vi "main.vi"() -> ()   [LabVIEW 2013]
doc: "使用该模板构建标准状态机设计模式。各状态执行代码并决定转移状态。将该设计模式与根据用户动作响应而执行代码的用户界面事件处理器模式相比较。同时将该设计模式与每段消息处理代码可以将零至多个新消息加入队列的队列消息处理器模式相比较。\n注：该模板的设计未遵守最新NI推荐的编程风格。请通过“创建项目”对话框（而不要采用该模板），创建基于项目的标准状态机模式的完整实现。"
uses:
  main.ctl
panel:
  in  "添加":bool
  in  "商店信息":cluster{"店名":string, "营业":bool, "位置":string}
  in  "树形":string(tree)
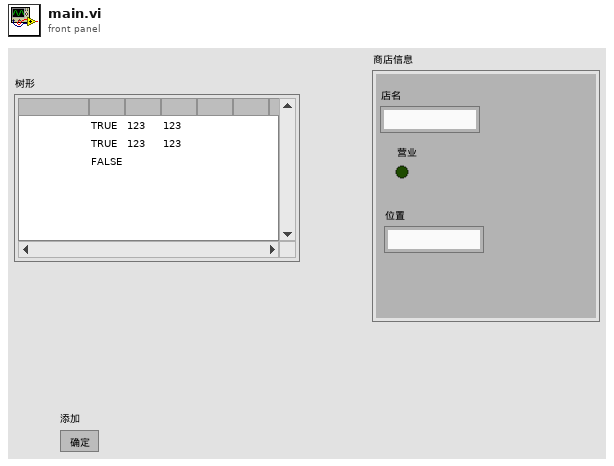
[diagram p1: front panel]
types:
  T1 = typedef "main.ctl" = enum16{"删除商店信息", "添加商店信息", "Initialize", "Stop"}
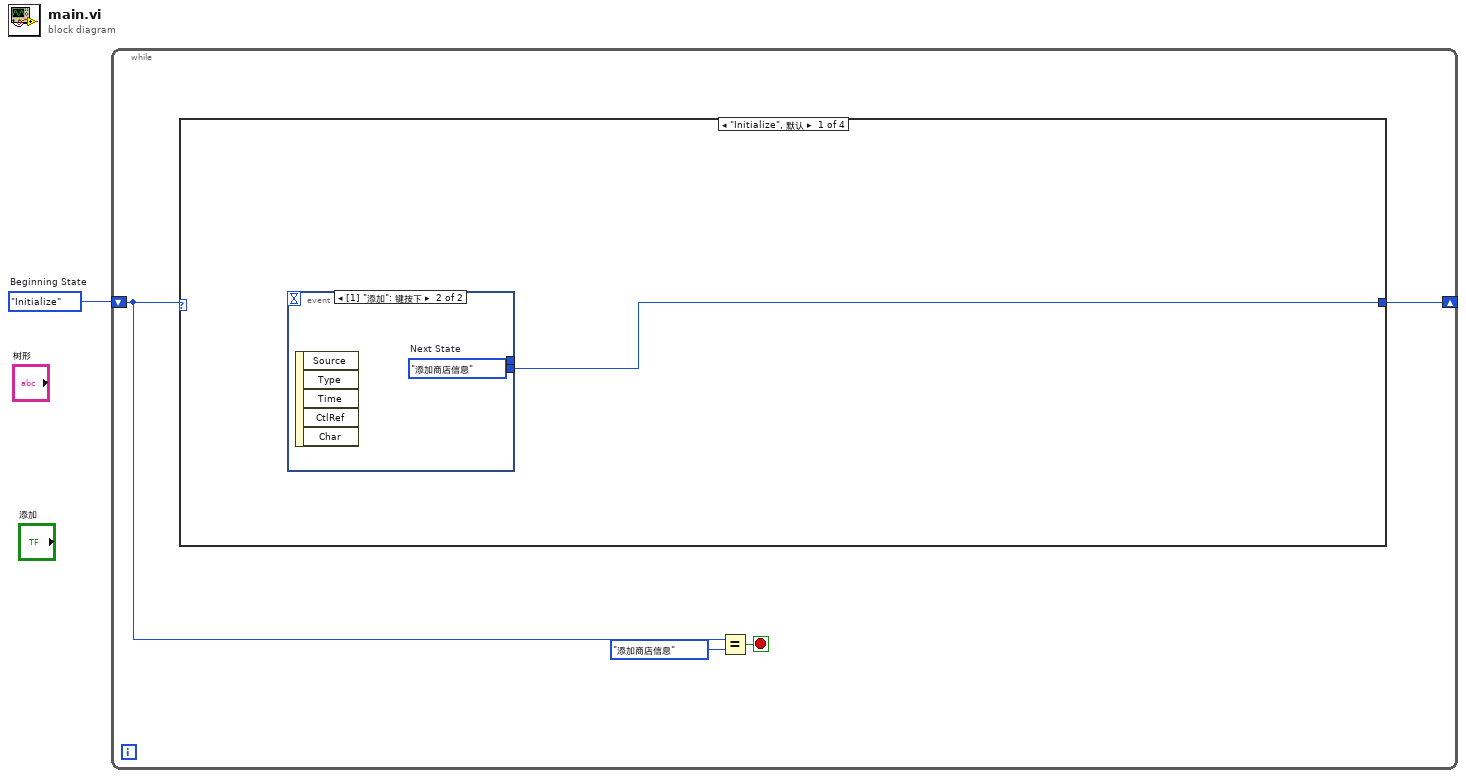
[diagram p0: block diagram]
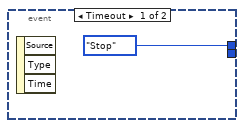
[diagram p2: hidden frame]
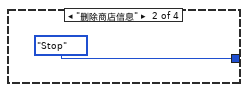
[diagram p3: hidden frame]
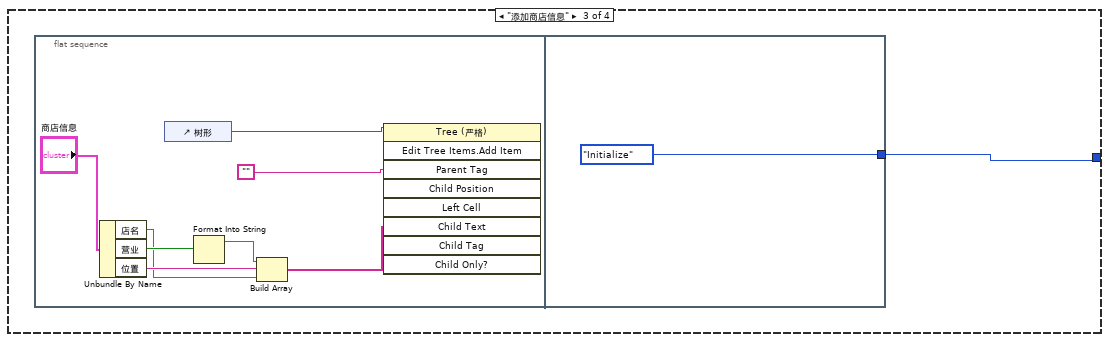
[diagram p4: hidden frame]
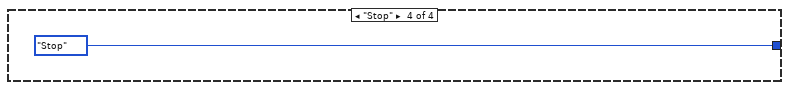
[diagram p5: hidden frame]
diagram:
  w1 = main."Initialize"  # Beginning State
  n1 = while {
    shift-right: [w2] -> _
    shift-left: w1 -> [w3]
    stop <- w5 stop-if-true
    n2 = case shown="\"Initialize\", 默认" w3 {
      tunnel: [w6 main."Stop" ("States") w10 main."Stop" ("Next State")] -> w2
      frame "Initialize", Default {
        n3 = event shown="[1] \"添加\": 键按下" {
          selector: _ -> [_ _]
          dyn-events: _ -> [_ _]
          timeout: _ -> [_ _]
          tunnel: [_ w8] -> w6
          tunnel: [main."Stop" ("States") _] -> _
          event Timeout {
            n4 = event-data() -> ()  [unwired: 1 in, 3 out]
          }
          event "添加": Key Down {
            w8 = main."添加商店信息"  # Next State
            n5 = event-data() -> ()  [unwired: 1 in, 5 out]
          }
        }
      }
      frame "删除商店信息" {
      }
      frame "添加商店信息" {
        n6 = flat-sequence {
          tunnel: [main."Initialize" ("States")] -> w10
          frame #0 {
            n7 = Unbundle By Name("商店信息") -> ("店名"=w11:string, "营业"=w16:bool, "位置"=w17:string)
            n8 = control-ref of="树形"() -> (w14:refnum<vi>)
            n9 = Format Into String(w16) -> (resulting string=w12:string)  [unwired: 3 in, 1 out]
            n10 = Build Array(w12, w17, w11) -> (w18:string[])
            n11 = invoke class="Tree (严格)" method="Edit Tree Items.Add Item"(reference=w14, "Parent Tag"="", "Child Text"=w18) -> ()  [unwired: 6 in, 9 out]
          }
          frame #1 {
          }
        }
      }
      frame "Stop" {
      }
    }
    n12 = Equal?(x=w3, y=main."添加商店信息" ("States")) -> (x = y?=w5:bool)
  }
